vi "ZCAN_InitCAN( I ).vi"(4 "error in (no error)":errorcluster caption="错误输入（无错误）", 5 "I系列初始化参数":T1, 6 "can_index":u32, 7 "device_hande":u32) -> (0 "error out":errorcluster caption="错误输出", 2 "can_index_handle":u32)   [LabVIEW 2018]
doc: "用于设置CAN通道的初始化参数。\n\n参数包括：波特率（自定义波特率）、滤波、工作模式；\n\n适用的设备：USBCAN-I、USBCAN-II、PCI9810、PCI9820、PCI5110、PCIe-9110I、PCI9820I、PCIE-9221、PCIe-9120I、PCI5121。"
uses:
  data_type/ZCAN_InitCAN_setting_I.ctl
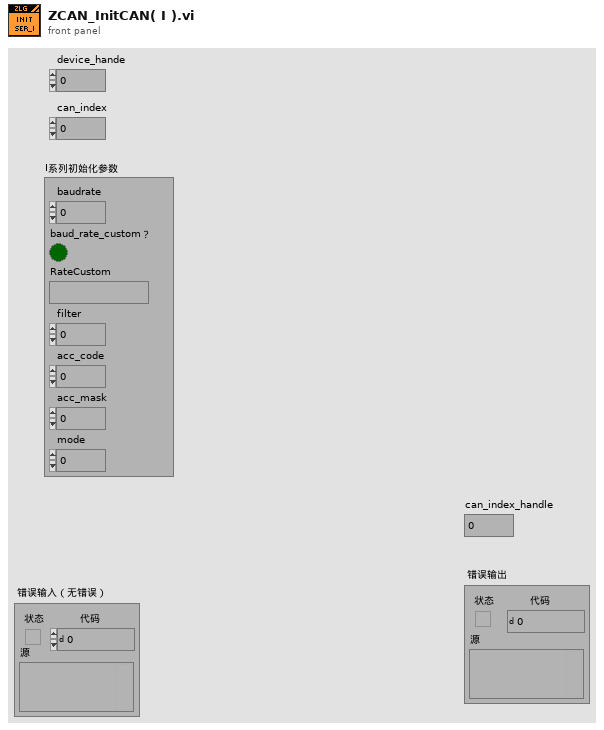
[diagram p1: front panel]
types:
  T1 = typedef "ZCAN_InitCAN_setting_I.ctl" = cluster{"baudrate":u32, "baud_rate_custom？":bool, "RateCustom":string, "filter":u8, "acc_code":u32, "acc_mask":u32, "mode":u8}
  T2 = cluster{"can_type":u32, "acc_code":u32, "acc_mask":u32, "can_type":u32, "filter":u8, "can_type":u8, "can_type":u8, "mode":u8}
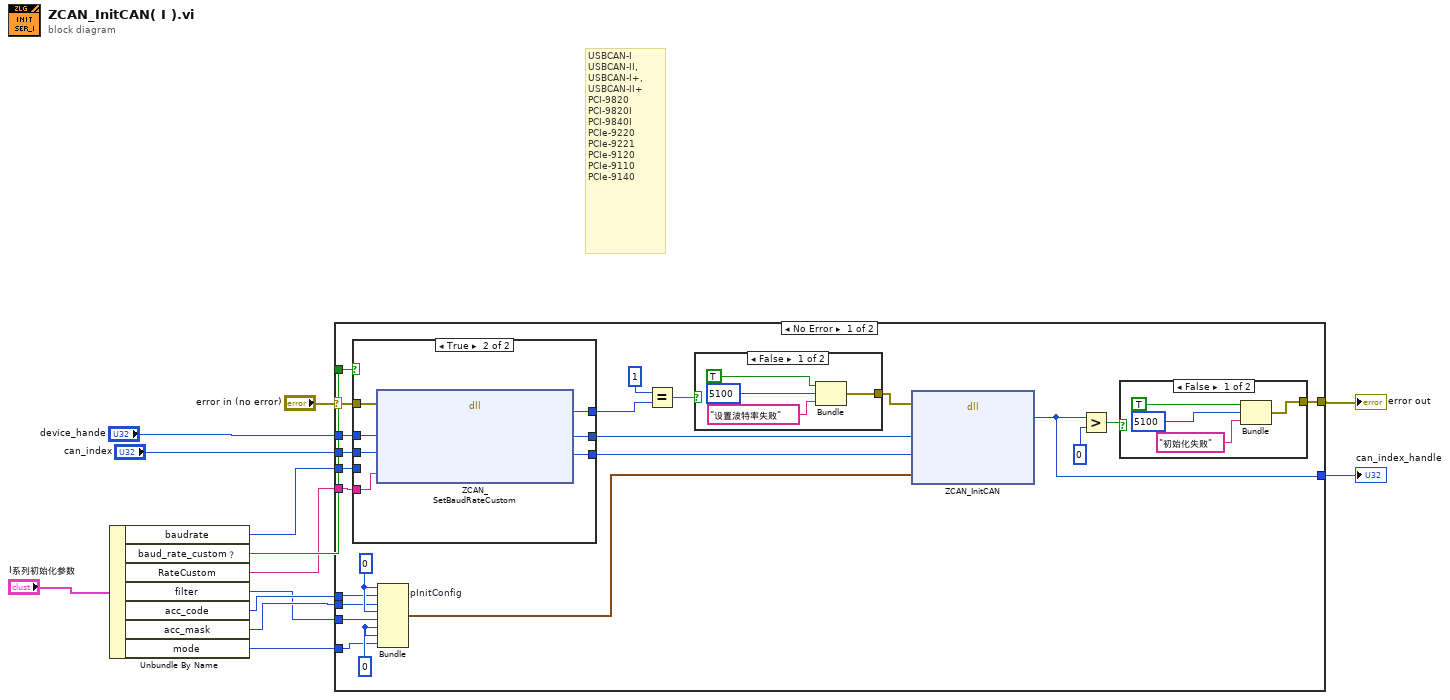
[diagram p0: block diagram]
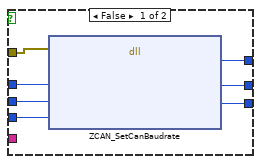
[diagram p4: hidden frame]
diagram:
  # "USBCAN-I\nUSBCAN-II,\nUSBCAN-I+,\nUSBCAN-II+ \nPCI-9820\nPCI-9820I\nPCI-9840I\nPCIe-9220 \nPCIe-9221\nPCIe-9120 \nPCIe-9110 \nPCIe-9140"
  n1 = Unbundle By Name("I系列初始化参数") -> ("baudrate"=w7:u32, "baud_rate_custom？"=w6:bool, "RateCustom"=w5:string, "filter"=w2:u8, "acc_code"=w4:u32, "acc_mask"=w3:u32, "mode"=w1:u8)
  n2 = case shown="No Error" "error in (no error)" {
    selector: "error in (no error)" -> [w31 w59]
    tunnel: [w18 w59] -> w12
    tunnel: w6 -> [w36 _]
    tunnel: "device_hande" -> [w35 _]
    tunnel: "can_index" -> [w34 _]
    tunnel: w7 -> [w33 _]
    tunnel: w5 -> [w32 _]
    tunnel: [w19 _] -> w11
    tunnel: w4 -> [w17 _]
    tunnel: w3 -> [w16 _]
    tunnel: w2 -> [w15 _]
    tunnel: w1 -> [w14 _]
    frame No Error {
      w26 = u8 0 ("can_type")
      w27 = u32 0 ("can_type")
      n3 = case shown="True" w36 {
        tunnel: w35 -> [w51 w58]
        tunnel: w34 -> [w50 w57]
        tunnel: w33 -> [w49 _]
        tunnel: w32 -> [_ w52]
        tunnel: [w47 w56] -> w30
        tunnel: [w46 w55] -> w29
        tunnel: w31 -> [w45 w54]
        tunnel: [w48 w53] -> w24
        frame False {
          n4 = dll-call lib="PTH2tabs CUsersadminDesktop'完善2020版本zlgcan_labview_20220510zlgcan_demo_CANET_UDPbinzlgcan_wrap.dll" fn="ZCAN_SetCanBaudrate"(error in=w45, "hDev"=w51, "can_index"=w50, "baudrate"=w49) -> ("return"=w48:u32, "hDev"=w47:u32, "can_index"=w46:u32)  [unwired: 3 in, 2 out]
        }
        frame True {
          n5 = dll-call lib="PTH2tabs CUsersadminDesktop'完善2020版本zlgcan_labview_20220510zlgcan_demo_CANET_UDPbinzlgcan_wrap.dll" fn="ZCAN_SetBaudRateCustom"(error in=w54, "device_handle"=w58, "can_index"=w57, "RateCustom"=w52) -> ("return"=w53:u32, "device_handle"=w56:u32, "can_index"=w55:u32)  [unwired: 3 in, 2 out]
        }
      }
      n6 = Bundle "pInitConfig"("can_type"=w27, "acc_code"=w17, "acc_mask"=w16, "can_type"=w27, "filter"=w15, "can_type"=w26, "can_type"=w26, "mode"=w14) -> (w28:T2)  [unwired: 1 in]
      n7 = Equal?(x=1, y=w24) -> (x = y?=w23:bool)
      n8 = case shown="False" w23 {
        tunnel: [w41 _] -> w22
        frame False {
          n9 = Bundle("status"=TRUE, "code"=5100, "消息"="设置波特率失败") -> (w41:cluster{"status":bool, "code":i32, "消息":string})  [unwired: 1 in]
        }
        frame True {
        }
      }
      n10 = dll-call lib="PTH2tabs CUsersadminDesktop'完善2020版本zlgcan_labview_20220510zlgcan_demo_CANET_UDPbinzlgcan_wrap.dll" fn="ZCAN_InitCAN"(error in=w22, "device_handle"=w30, "can_index"=w29, "pInitConfig"=w28) -> ("can_handle"=w19:u32)  [unwired: 5 in, 2 out]
      n11 = Greater?(x=w19, y=0) -> (0:w20:bool)
      n12 = case shown="False" w20 {
        tunnel: [w37 _] -> w18
        frame False {
          n13 = Bundle("status"=TRUE, "code"=5100, "消息"="初始化失败") -> (w37:cluster{"status":bool, "code":i32, "消息":string})  [unwired: 1 in]
        }
        frame True {
        }
      }
    }
    frame Error {
    }
  }
  "error out" <- w12
  "can_index_handle" <- w11
